vi "DAC Configure.vi"(8 "error in":errorcluster, 11 "DAC HeatFlow AIV in":refnum<class "DAC HeatFlow AIV.lvclass">) -> (0 "error out":errorcluster, 3 "DAC HeatFlow AIV out":refnum<class "DAC HeatFlow AIV.lvclass">)   [LabVIEW 2019, in "DAC.lvlib" / "DAC HeatFlow AIV.lvclass"]
uses:
  DAC HeatFlow AIV.lvclass
  C:/Users/krio/Documents/LV_Projects/test-stand/App/DAC/DAC.lvclass
  DAC.lvclass/DAC.ctl
  DAC HeatFlow AIV.lvclass/DAC HeatFlow AIV.ctl
  <vilib>/Utility/error.llb/Error Cluster From Error Code.vi
  <vilib>/DAQmx/create/channels.llb/DAQmx Create Channel (AI-Voltage-Basic).vi
  <vilib>/ErrorRing/Error Ring.xnode
  DAC.lvclass
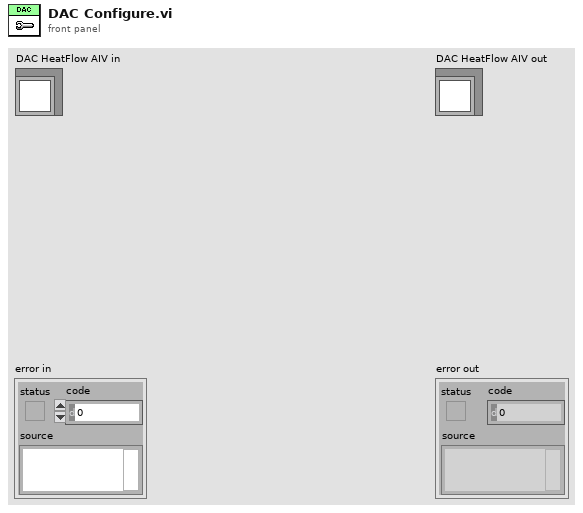
[diagram p1: front panel]
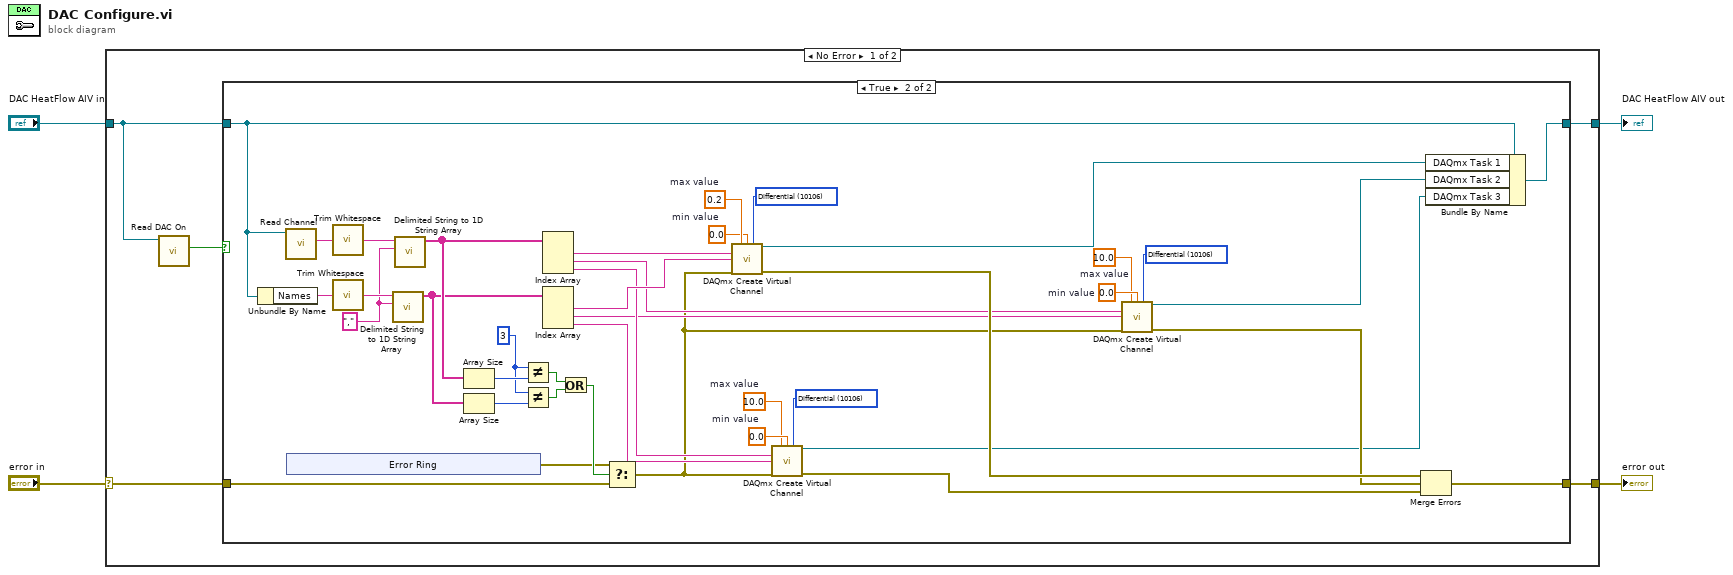
[diagram p0: block diagram]
diagram:
  n1 = case shown="No Error" "error in" {
    selector: "error in" -> [w6 w57]
    tunnel: [w5 w57] -> w4
    tunnel: [w7 w56] -> w3
    tunnel: "DAC HeatFlow AIV in" -> [w9 w56]
    frame No Error {
      n2 = call "Read DAC On.vi"("DAC in"=w9) -> ("DAC On"=w8:bool)  [unwired: 8 in, 2 out]
      n3 = case shown="True" w8 {
        tunnel: w9 -> [w11 w50]
        tunnel: [w11 w51] -> w7
        tunnel: w6 -> [w10 w33]
        tunnel: [w10 w12] -> w5
        frame False {
        }
        frame True {
          w22 = 10106 items=["Default"=-1, "RSE"=10083, "NRSE"=10078, "Differential"=10106, "Pseudodifferential"=12529] ("input terminal configuration")
          w21 = 0.0  # min value
          w20 = 10.0  # max value
          w27 = 10106 items=["Default"=-1, "RSE"=10083, "NRSE"=10078, "Differential"=10106, "Pseudodifferential"=12529] ("input terminal configuration")
          w26 = 0.0  # min value
          w25 = 10.0  # max value
          w37 = 3 ("x")
          w40 = "," ("delimiter")
          w45 = 10106 items=["Default"=-1, "RSE"=10083, "NRSE"=10078, "Differential"=10106, "Pseudodifferential"=12529] ("input terminal configuration")
          w46 = 0.0  # min value
          w47 = 0.2  # max value
          n4 = Unbundle By Name(w50) -> ("Names"=w43:string)
          n5 = call "Read Channel.vi"("DAC in"=w50) -> ("Channel"=w44:string)  [unwired: 8 in, 2 out]
          n6 = xnode "Error Ring"() -> ("error out"=w32:errorcluster)
          n7 = call <vilib>:"Trim Whitespace.vi"("string"=w44) -> ("trimmed string"=w42:string)  [unwired: 1 in]
          n8 = call <vilib>:"Trim Whitespace.vi"("string"=w43) -> ("trimmed string"=w41:string)  [unwired: 1 in]
          n9 = call <vilib>:"Delimited String to 1D String Array.vi"("delimiter"=w40, "delimited string"=w41) -> ("string array"=w30:string[])  [unwired: 9 in]
          n10 = call <vilib>:"Delimited String to 1D String Array.vi"("delimiter"=w40, "delimited string"=w42) -> ("string array"=w31:string[])  [unwired: 9 in]
          n11 = Array Size(array=w31) -> (size(s)=w39:i32)
          n12 = Array Size(array=w30) -> (size(s)=w38:i32)
          n13 = Not Equal?(x=w37, y=w39) -> (x != y?=w36:bool)
          n14 = Not Equal?(x=w37, y=w38) -> (x != y?=w35:bool)
          n15 = Index Array(array=w31) -> (element #1=w29:string, element #2=w17:string, element #3=w16:string)  [unwired: 3 in]
          n16 = Index Array(array=w30) -> (element #1=w28:string, element #2=w15:string, element #3=w14:string)  [unwired: 3 in]
          n17 = Or(x=w36, y=w35) -> (x .or. y?=w34:bool)
          n18 = Select(t=w32, s=w34, f=w33) -> (s? t:f=w13:errorcluster)
          n19 = call-poly <vilib>:"DAQmx Create Virtual Channel.vi"("maximum value"=w47, "minimum value"=w46, "input terminal configuration"=w45, "physical channels"=w29, "name to assign"=w28, "error in"=w13) -> ("task out"=w49:refnum<k21>, "error out"=w48:errorcluster)  [unwired: 8 in]
          n20 = call-poly <vilib>:"DAQmx Create Virtual Channel.vi"("maximum value"=w20, "minimum value"=w21, "input terminal configuration"=w22, "physical channels"=w16, "name to assign"=w14, "error in"=w13) -> ("task out"=w18:refnum<k21>, "error out"=w19:errorcluster)  [unwired: 8 in]
          n21 = call-poly <vilib>:"DAQmx Create Virtual Channel.vi"("maximum value"=w25, "minimum value"=w26, "input terminal configuration"=w27, "physical channels"=w17, "name to assign"=w15, "error in"=w13) -> ("task out"=w23:refnum<k21>, "error out"=w24:errorcluster)  [unwired: 8 in]
          n22 = Merge Errors(w48, w24, w19) -> (w12:errorcluster)
          n23 = Bundle By Name(cluster=w50, "DAQmx Task 1"=w49, "DAQmx Task 2"=w23, "DAQmx Task 3"=w18) -> (w51:refnum<class "DAC HeatFlow AIV.lvclass">)
        }
      }
    }
    frame Error {
    }
  }
  "error out" <- w4
  "DAC HeatFlow AIV out" <- w3
